vi "Proyecto TOOLKIT.vi"() -> ()   [LabVIEW 2013]
uses:
  <vilib>/userdefined/High Color/IMAQdx.ctl
  <vilib>/vision/driver/NI_Vision_Acquisition_Software.lvlib
  <vilib>/vision/NI_Vision_Development_Module.lvlib
  <vilib>/LabVIEW Interface for Arduino/LabVIEW Interface for Arduino.lvlib
panel:
  in  "Centro de Y":dbl
  in  "Centro de X":dbl
  out "Pos. Servo Y":dbl
  out "Pos. Servo X":dbl
  out "Objeto Detectado":bool
  out "X":bool
  out "-Y":bool
  out "-X":bool
  out "Y":bool
  out "Valor de Y":sgl
  out "Valor de X":sgl
  in  "Color Plane":i32(ring)=1 items=["Red", "Green", "Blue", "Hue", "Saturation", "Luminance", "Value", "Intensity"]
  in  "stop":bool
  out "Image":T1(plugin-control)
  in  "Settings":T2={"Algorithm"=2, "Number of Matches Requested"=1, "Minimum Match Score"=800.0, "SubPixel Accuracy"=TRUE, "Rotation Angle Ranges"=[], "Show Search Area"=FALSE, "Show Result"=TRUE} {"Rotation Angle Ranges"."End" format="%.1f"; "Rotation Angle Ranges"."Start" format="%.1f"; "Minimum Match Score" min=0 max=1000 format="%.2f"; "Number of Matches Requested" min=1; "Algorithm" items=["All", "Low Discrepancy Sampling", "Grayscale Value Pyramid", "Gradients Pyramid"]}
  in  "Search Rect":T3={"Left"=0, "Top"=0, "Right"=2147483647, "Bottom"=2147483647, "Rotation"=0.0} {"Rotation" format="%.2f"; "Left" scale=0.0..1024.0; "Right" scale=0.0..1024.0}
  in  "File Path":path
  # "Valores en servo X 45°\nSi servo>45°=Abajo\nSi servo<45°=Arriba"
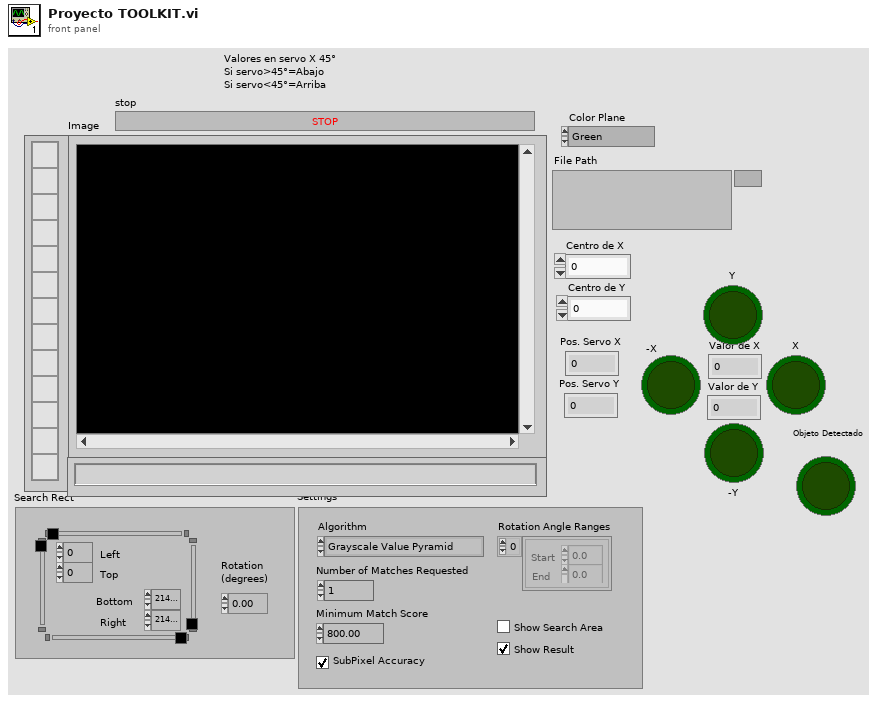
[diagram p1: front panel]
types:
  T1 = typedef "IMAQ Image.ctl" = refnum<image>
  T2 = cluster{"Algorithm":i32, "Number of Matches Requested":i32, "Minimum Match Score":sgl, "SubPixel Accuracy":bool, "Rotation Angle Ranges":cluster{"Start":sgl, "End":sgl}[], "Show Search Area":bool, "Show Result":bool}
  T3 = typedef "IMAQ Rectangle" = cluster{"Left":i32, "Top":i32, "Right":i32, "Bottom":i32, "Rotation":dbl}
  T4 = typedef "IMAQdx.ctl" = refnum<k21>
  T5 = typedef "LabVIEW Interface for Arduino.lvlib/Arduino Resource.ctl" = cluster{"VISA resource":refnum<visa-resource-name>, "Board Type":T6, "Connection Type":enum8{"USB / Serial"}, "Bytes Per Packet (15)":u8}
  T6 = typedef "LabVIEW Interface for Arduino.lvlib/Board Type.ctl" = enum16{"Uno", "Dimuelanove w/Atmega 328", "Mega 2560"}
  T7 = cluster{"Position":cluster{"x":sgl, "y":sgl}, "Angle":sgl, "Scale":sgl, "Score":sgl, "Bounding Box":cluster{"x":sgl, "y":sgl}[]}[]
  T8 = cluster{"Matches (pixel)[0]":cluster{"Position":cluster{"x":sgl, "y":sgl}, "Angle":sgl, "Scale":sgl, "Score":sgl, "Bounding Box":cluster{"x":sgl, "y":sgl}[]}, "Matches (pixel)[1]":cluster{"Position":cluster{"x":sgl, "y":sgl}, "Angle":sgl, "Scale":sgl, "Score":sgl, "Bounding Box":cluster{"x":sgl, "y":sgl}[]}, "Matches (pixel)[2]":cluster{"Position":cluster{"x":sgl, "y":sgl}, "Angle":sgl, "Scale":sgl, "Score":sgl, "Bounding Box":cluster{"x":sgl, "y":sgl}[]}, "Matches (pixel)[3]":cluster{"Position":cluster{"x":sgl, "y":sgl}, "Angle":sgl, "Scale":sgl, "Score":sgl, "Bounding Box":cluster{"x":sgl, "y":sgl}[]}, "Matches (pixel)[4]":cluster{"Position":cluster{"x":sgl, "y":sgl}, "Angle":sgl, "Scale":sgl, "Score":sgl, "Bounding Box":cluster{"x":sgl, "y":sgl}[]}, "Matches (pixel)[5]":cluster{"Position":cluster{"x":sgl, "y":sgl}, "Angle":sgl, "Scale":sgl, "Score":sgl, "Bounding Box":cluster{"x":sgl, "y":sgl}[]}, "Matches (pixel)[6]":cluster{"Position":cluster{"x":sgl, "y":sgl}, "Angle":sgl, "Scale":sgl, "Score":sgl, "Bounding Box":cluster{"x":sgl, "y":sgl}[]}, "Matches (pixel)[7]":cluster{"Position":cluster{"x":sgl, "y":sgl}, "Angle":sgl, "Scale":sgl, "Score":sgl, "Bounding Box":cluster{"x":sgl, "y":sgl}[]}, "Matches (pixel)[8]":cluster{"Position":cluster{"x":sgl, "y":sgl}, "Angle":sgl, "Scale":sgl, "Score":sgl, "Bounding Box":cluster{"x":sgl, "y":sgl}[]}}
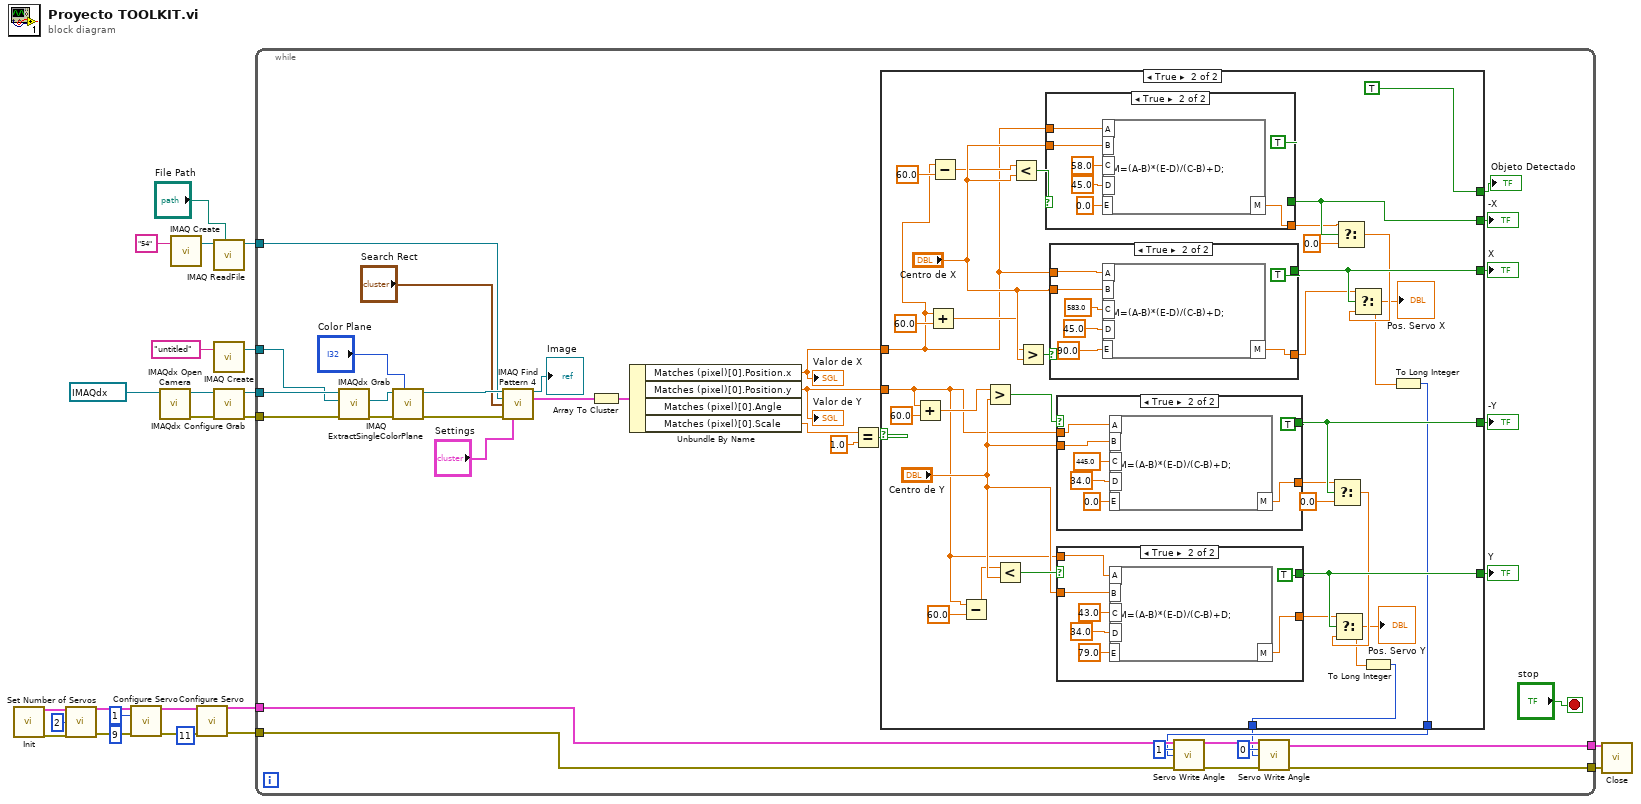
[diagram p0: block diagram]
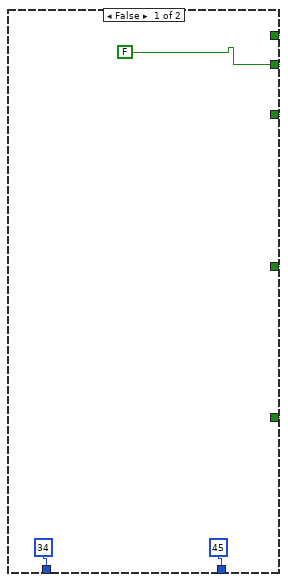
[diagram p2: hidden frame]
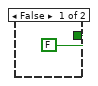
[diagram p3: hidden frame]
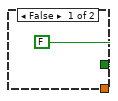
[diagram p4: hidden frame]
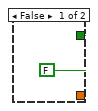
[diagram p5: hidden frame]
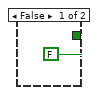
[diagram p6: hidden frame]
diagram:
  n1 = call <vilib>:"Init.vi"() -> ("Arduino Resource"=w14:T5, "error out"=w13:errorcluster)  [unwired: 18 in]
  n2 = call <vilib>:"Set Number of Servos.vi"("Arduino Resource"=w14, "Number Of Servos (1)"=u8 2, "error in"=w13) -> ("Arduino Resource"=w11:T5, "error out"=w10:errorcluster)  [unwired: 11 in]
  n3 = call <vilib>:"Configure Servo.vi"("Arduino Resource"=w11, "Servo Number (0)"=u8 1, "DIO Pin (2)"=u8 9, "error in"=w10) -> ("Arduino Resource"=w7:T5, "error out"=w6:errorcluster)  [unwired: 10 in]
  n4 = call <vilib>:"IMAQdx Open Camera.vi"("Session In"=T4 "cam1") -> ("error out"=w25:errorcluster, "Session Out"=w24:T4)  [unwired: 9 in]
  n5 = call "IMAQ Create"("Image Name"="54") -> ("New Image"=w17:T1)  [unwired: 4 in, 1 out]
  n6 = call <vilib>:"Configure Servo.vi"("Arduino Resource"=w7, "DIO Pin (2)"=u8 11, "error in"=w6) -> ("Arduino Resource"=w4:T5, "error out"=w3:errorcluster)  [unwired: 11 in]
  n7 = call "IMAQ ReadFile"("File Path"="File Path", "Image"=w17) -> ("Image Out"=w16:T1)  [unwired: 5 in, 4 out]
  n8 = call "IMAQ Create"("Image Name"="untitled") -> ("New Image"=w19:T1)  [unwired: 4 in, 1 out]
  n9 = call <vilib>:"IMAQdx Configure Grab.vi"("error in"=w25, "Session In"=w24) -> ("error out"=w22:errorcluster, "Session Out"=w23:T4)  [unwired: 8 in]
  n10 = while {
    tunnel: w23 -> [w60]
    tunnel: w22 -> [w59]
    tunnel: w19 -> [w55]
    tunnel: w16 -> [w53]
    tunnel: w4 -> [w35]
    tunnel: w3 -> [w34]
    tunnel: [w30] -> w2
    tunnel: [w29] -> w1
    stop <- "stop" stop-if-true
    n11 = call <vilib>:"IMAQdx Grab.vi"("error in"=w59, "Image In"=w55, "Session In"=w60) -> ("error out"=w58:errorcluster, "Image Out"=w54:T1)  [unwired: 5 in, 2 out]
    n12 = call "IMAQ ExtractSingleColorPlane"("Color Plane"="Color Plane", "error in (no error)"=w58, "Image Src"=w54) -> ("error out"=w56:errorcluster, "Image Dst Out"=w57:T1)  [unwired: 7 in]
    n13 = call "IMAQ Find Pattern 4"("Image"=w57, "Template"=w53, "Search Rect"="Search Rect", "error in"=w56, "Settings"="Settings") -> ("Image Out"=→"Image":T1, "Matches (pixel)"=w47:T7)  [unwired: 4 in, 5 out]
    n14 = Array To Cluster(array=w47) -> (cluster=w48:T8)
    n15 = Unbundle By Name(w48) -> ("Matches (pixel)[0].Position.x"=w46:sgl, "Matches (pixel)[0].Position.y"=w45:sgl, "Matches (pixel)[0].Scale"=w44:sgl)  [unwired: 1 out]
    "Valor de X" <- w46
    "Valor de Y" <- w45
    n16 = Equal?(x=w44, y=sgl 1.0) -> (x = y?=w42:bool)
    n17 = case shown="True" w42 {
      tunnel: w46 -> [_ w69]
      tunnel: w45 -> [_ w64]
      tunnel: [w63 TRUE] -> w41
      tunnel: [w63 w88] -> w40
      tunnel: [w63 w91] -> w39
      tunnel: [w63 w85] -> w38
      tunnel: [w63 w82] -> w37
      tunnel: [45 w77] -> w27
      tunnel: [34 w75] -> w26
      frame False {
        w63 = FALSE
      }
      frame True {
        n18 = Add(x=w64, y=60.0) -> (x+y=w66:dbl)
        n19 = Add(x=w69, y=60.0) -> (x+y=w73:dbl)
        n20 = Subtract(x=w69, y=60.0) -> (x-y=w71:dbl)
        n21 = Subtract(x=w64, y=60.0) -> (x-y=w68:dbl)
        n22 = Greater?(x=w66, y="Centro de Y") -> (0:w95:bool)
        n23 = Less?(x=w68, y="Centro de Y") -> (x < y?=w93:bool)
        n24 = Less?(x=w71, y="Centro de X") -> (x < y?=w94:bool)
        n25 = Greater?(x=w73, y="Centro de X") -> (0:w96:bool)
        n26 = case shown="True" w94 {
          tunnel: [FALSE TRUE] -> w91
          tunnel: "Centro de X" -> [_ w110]
          tunnel: w69 -> [_ w109]
          tunnel: [_ w106] -> w90
          frame False {
          }
          frame True {
            n27 = formula code="M=(A-B)*(E-D)/(C-B)+D;"("A"=w109, "B"=w110, "C"=58.0 ("input variable"), "D"=45.0 ("input variable"), "E"=0.0 ("input variable")) -> ("M"=w106:dbl)
          }
        }
        n28 = case shown="True" w96 {
          tunnel: [FALSE TRUE] -> w88
          tunnel: w69 -> [_ w124]
          tunnel: "Centro de X" -> [_ w123]
          tunnel: [_ w122] -> w87
          frame False {
          }
          frame True {
            n29 = formula code="M=(A-B)*(E-D)/(C-B)+D;"("A"=w124, "B"=w123, "C"=583.0 ("input variable"), "D"=45.0 ("input variable"), "E"=90.0 ("input variable")) -> ("M"=w122:dbl)
          }
        }
        n30 = case shown="True" w95 {
          tunnel: [FALSE TRUE] -> w85
          tunnel: "Centro de Y" -> [_ w118]
          tunnel: [_ w115] -> w84
          tunnel: w64 -> [_ w114]
          frame False {
          }
          frame True {
            n31 = formula code="M=(A-B)*(E-D)/(C-B)+D;"("A"=w114, "B"=w118, "C"=445.0 ("input variable"), "D"=34.0 ("input variable"), "E"=0.0 ("input variable")) -> ("M"=w115:dbl)
          }
        }
        n32 = case shown="True" w93 {
          tunnel: [FALSE TRUE] -> w82
          tunnel: "Centro de Y" -> [_ w102]
          tunnel: w64 -> [_ w101]
          tunnel: [_ w98] -> w81
          frame False {
          }
          frame True {
            n33 = formula code="M=(A-B)*(E-D)/(C-B)+D;"("A"=w101, "B"=w102, "C"=43.0 ("input variable"), "D"=34.0 ("input variable"), "E"=79.0 ("input variable")) -> ("M"=w98:dbl)
          }
        }
        n34 = Select(t=w84, s=w85, f=0.0) -> (s? t:f=w80:dbl)
        n35 = Select(t=w81, s=w82, f=w80) -> (s? t:f=w76:dbl)
        "Pos. Servo Y" <- w76
        n36 = Select(t=w90, s=w91, f=0.0) -> (s? t:f=w86:dbl)
        n37 = Select(t=w87, s=w88, f=w86) -> (s? t:f=w78:dbl)
        "Pos. Servo X" <- w78
        n38 = To Long Integer(number=w76) -> (32bit integer=w75:i32)
        n39 = To Long Integer(number=w78) -> (32bit integer=w77:i32)
      }
    }
    "Objeto Detectado" <- w41
    "X" <- w40
    "-X" <- w39
    "Y" <- w37
    "-Y" <- w38
    n40 = call <vilib>:"Servo Write Angle.vi"("Arduino Resource"=w35, "Servo Number"=u8 1, "Angle (Degrees)"=w27, "error in"=w34) -> ("Arduino Resource"=w32:T5, "error out"=w31:errorcluster)  [unwired: 10 in]
    n41 = call <vilib>:"Servo Write Angle.vi"("Arduino Resource"=w32, "Servo Number"=u8 0, "Angle (Degrees)"=w26, "error in"=w31) -> ("Arduino Resource"=w30:T5, "error out"=w29:errorcluster)  [unwired: 10 in]
  }
  n42 = call <vilib>:"Close.vi"("Arduino Resource"=w2, "error in"=w1) -> ()  [unwired: 13 in, 1 out]
